vi "Continuous Serial Write and Read_ET_Edited.vi"() -> ()   [LabVIEW 2024]
doc: "This example performs writes and reads on a serial port, as directed by the user. You can press the Write and Read buttons, and change the Read Count, while the example is running.\n\nThe parameters set for the serial port must match the parameters of the connected instrument or device. In this example, the Read Count parameter specifies the number of bytes that the serial port reads. If there were more bytes at the port than the specified number, those bytes would not be read. If there were less bytes at the port than the specified number, you would receive a timeout error.\n\nThis example expands upon the flow control options for XON and XOFF, allowing the user to choose those control characters. Also, the user can enable or disable a termination character. Some devices require a termination character in order to identify the end of command strings. Some devices send a termination character to signify the end of data to be read. This example shows how you can end the Read operation once a termination character is detected in the buffer and/or append a termination character at the end of the Write data."
uses:
  support/Serial - Settings.ctl
  support/Serial - XON-XOFF Characters.ctl
  support/Serial - ASCII Characters.ctl
  <vilib>/Instr/_visa.llb/VISA Configure Serial Port (Instr).vi
panel:
  out "return count":u32
  in  "Stop":bool
  in  "Commands":string[](array[string])=["*RST", "SYST:ZCH ON", "FUNC \"CURR\"", "SYST:ZCOR ON", "CURR:RANG:AUTO ON", "SYST:ZCH OFF", "READ?", ""]
  in  "Termination Character":u8=10 format="%.0x"
  in  "End Write on Termination Character?":bool=TRUE
  in  "Read Count":u32=1000
  out "Response":string
  in  "Write":bool
  in  "Read":bool
  in  "XON/XOFF Characters":T1={"XON"=enum."DC1", "XOFF"=enum."DC3"}
  in  "Serial Settings":T3={"baud rate"=9600, "data bits"=8, "parity"=enum."None", "stop bits"=10, "flow control"=0} {"flow control" items=["None"=0, "XON/XOFF"=1, "RTS/CTS"=2, "DTR/DSR"=4]; "stop bits" items=["1.0"=10, "1.5"=15, "2.0"=20]; "data bits" min=5 max=8 step=1; "baud rate" items=["75"=75, "110"=110, "134"=134, "150"=150, "300"=300, "600"=600, "1200"=1200, "1800"=1800, "2400"=2400, "4800"=4800, "7200"=7200, "9600"=9600, "14400"=14400, "19200"=19200, "28800"=28800, "38400"=38400, "56000"=56000, "57600"=57600, "115200"=115200, "128000"=128000, "230400"=230400]}
  in  "End Read on Termination Character?":bool=TRUE
  in  "VISA resource name":refnum<visa-resource-name>="COM1"
  # "Overview: Demonstrates the use of the VISA functions to write commands to and read responses from a serial instrument continuously in a loop.\nRequirements: NI-VISA Driver\nInstructions:\n1. Run the VI.\n2. Specify a Command and click the Write button.\n3. Read a Response by clicking the Read button.\n4. Click Stop to stop the VI."
  # "0xA is equivalent to a '\\n' character, which is a line feed."
  # "Multi-Commands can be given in one command if seperated by semicolons"
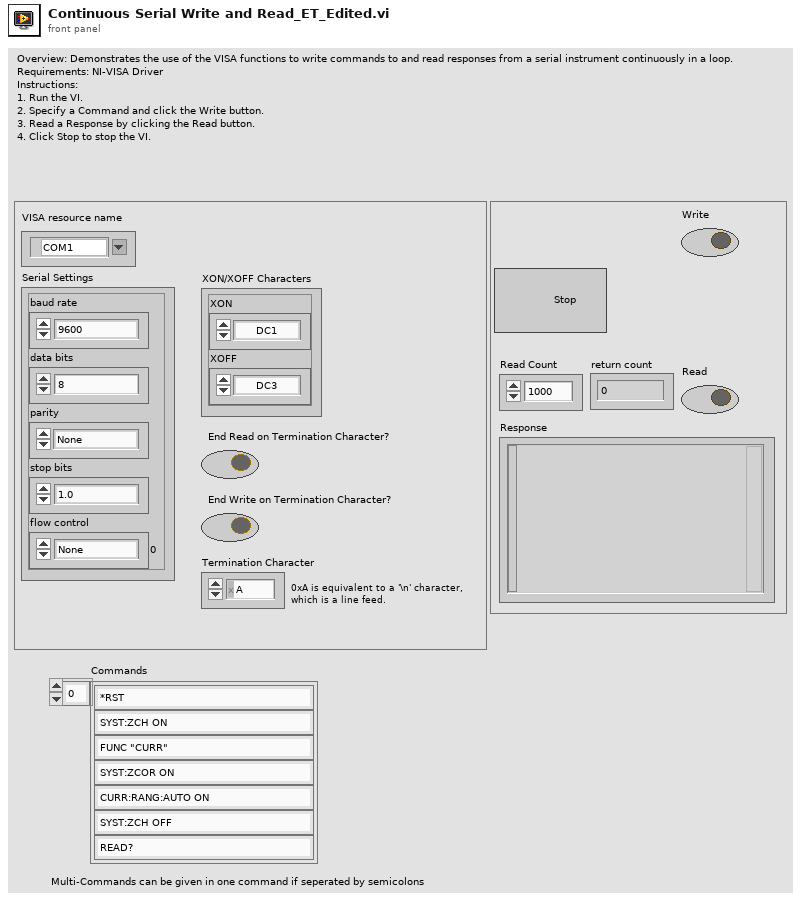
[diagram p1: front panel]
types:
  T1 = typedef "Serial - XON-XOFF Characters.ctl" = cluster{"XON":T2, "XOFF":T2}
  T2 = typedef "Serial - ASCII Characters.ctl" = enum16{"NUL", "SOH", "STX", "ETX", "EOT", "ENQ", "ACK", "BEL", "BS", "HT", "LF", "VT", "FF", "CR", "SO", "SI", "DLE", "DC1", "DC2", "DC3", "DC4", "NAK", "SYN", "ETB", "CAN", "EM", "SUB", "ESC", "FS", "GS", "RS", "US", "SP", "!", "\"", "#", "$", "%", "&", "'", "(", ")", "*", "+", ",", "- (-)", ".", "/", "0", "1", "2", "3", "4", "5", "6", "7", "8", "9", ":", ";", "<", "=", ">", "?", "@", "A", "B", "C", "D", "E", "F", "G", "H", "I", "J", "K", "L", "M", "N", "O", "P", "Q", "R", "S", "T", "U", "V", "W", "X", "Y", "Z", "[", "\\", "]", "^", "_", "`", "a", "b", "c", "d", "e", "f", "g", "h", "i", "j", "k", "l", "m", "n", "o", "p", "q", "r", "s", "t", "u", "v", "w", "x", "y", "z", "{", "|", "}", "~"}
  T3 = typedef "Serial - Settings.ctl" = cluster{"baud rate":u32, "data bits":u16, "parity":enum16{"None", "Odd", "Even", "Mark", "Space"}, "stop bits":u16, "flow control":u16}
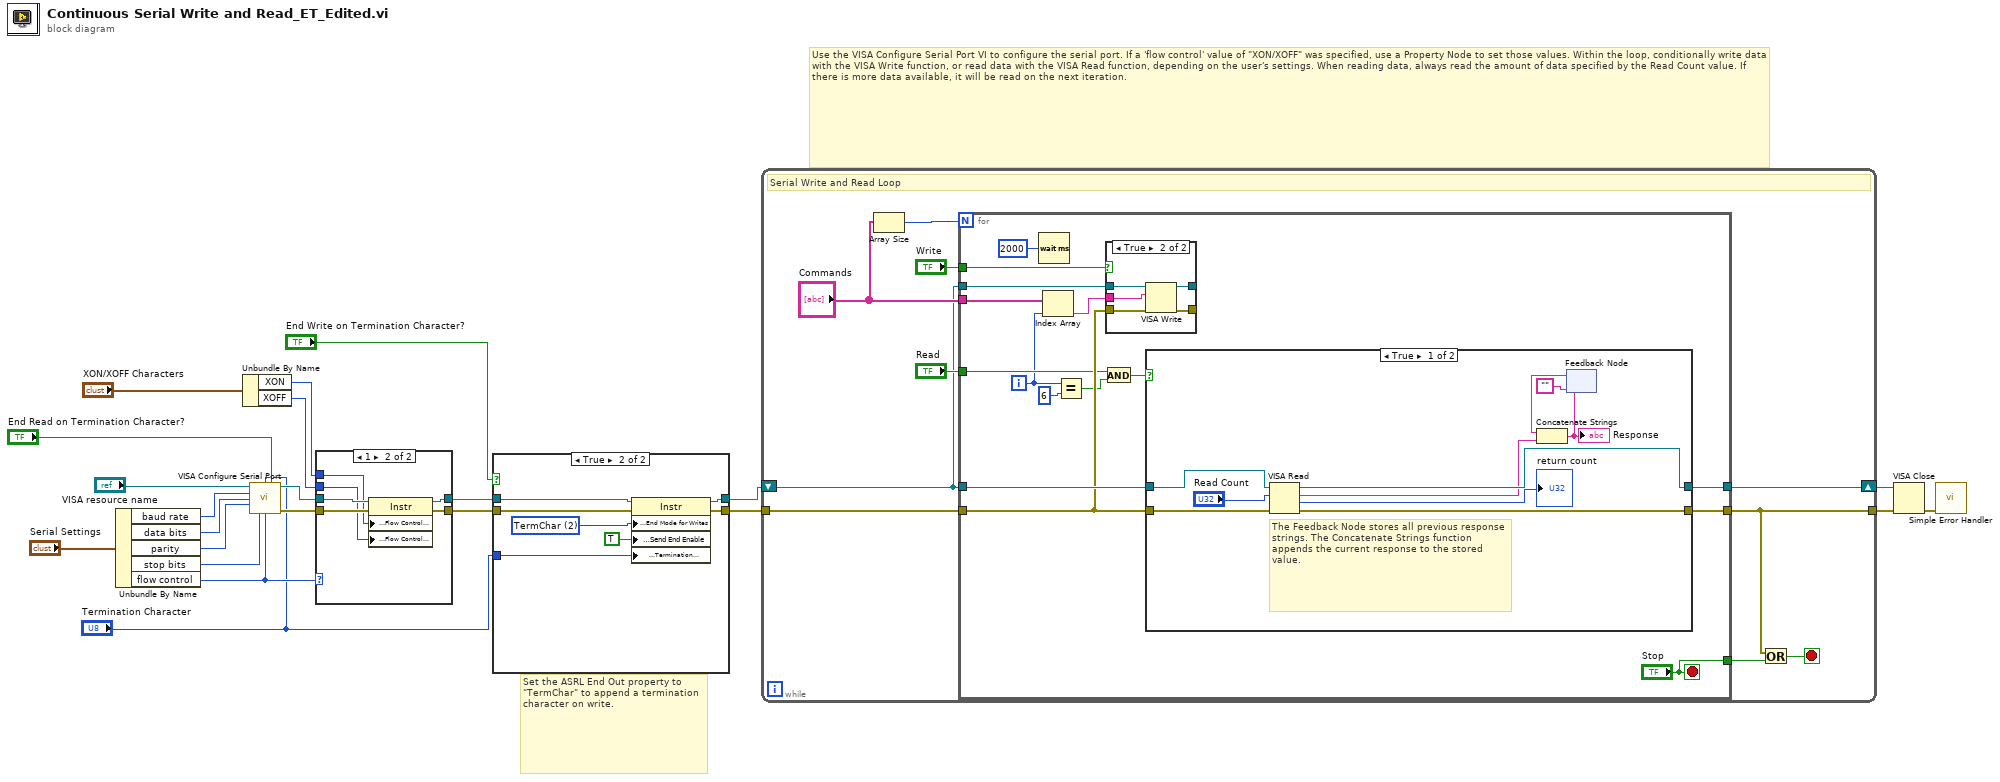
[diagram p0: block diagram]
diagram:
  # "Set the ASRL End Out property to \"TermChar\" to append a termination character on write."
  # "Use the VISA Configure Serial Port VI to configure the serial port. If a 'flow control' value of \"XON/XOFF\" was specified, use a Property Node to set those values. Within the loop, conditionally write data with the VISA Write function, or read data with the VISA Read function, depending on the user's settings. When reading data, always read the amount of data specified by the Read Count value. If there is more data available, it will be read on the next iteration."
  n1 = Unbundle By Name("Serial Settings") -> ("baud rate"=w15:u32, "data bits"=w16:u16, "parity"=w17:enum16{"None", "Odd", "Even", "Mark", "Space"}, "stop bits"=w18:u16, "flow control"=w9:u16)
  n2 = Unbundle By Name("XON/XOFF Characters") -> ("XON"=w8:T2, "XOFF"=w7:T2)
  n3 = call-poly "VISA Configure Serial Port"("VISA resource name"="VISA resource name", "termination char\n(0xA = '\\n' = LF)"="Termination Character", "Enable Termination\nChar (T)"="End Read on Termination Character?", "baud rate (9600)"=w15, "data bits (8)"=w16, "parity (0:none)"=w17, "stop bits (10: 1 bit)"=w18, "flow control (0:none)"=w9) -> ("VISA resource name out"=w19:refnum<visa-resource-name>, "error out"=w20:errorcluster)  [unwired: 2 in, 4 out]
  n4 = case shown="1" w9 {
    tunnel: [w23 w30] -> w6
    tunnel: [w24 w29] -> w4
    tunnel: w20 -> [w23 w28]
    tunnel: w19 -> [w24 w27]
    tunnel: w8 -> [_ w26]
    tunnel: w7 -> [_ w25]
    frame Default {
    }
    frame 1 {
      n5 = property class="Instr"(reference=w27, error in=w28, "Serial Settings:Flow Control XON Character"=w26, "Serial Settings:Flow Control XOFF Character"=w25) -> (reference out=w29:refnum<visa-resource-name>, error out=w30:errorcluster)
    }
  }
  n6 = case shown="True" "End Write on Termination Character?" {
    tunnel: w4 -> [w31 w39]
    tunnel: w6 -> [w32 w38]
    tunnel: [w31 w37] -> w3
    tunnel: [w32 w36] -> w5
    tunnel: "Termination Character" -> [_ w34]
    frame False {
    }
    frame True {
      w35 = u16 2 items=["None", "LastBit", "TermChar", "Break"] ("Serial Settings:Serial End Mode for Writes")
      n7 = property class="Instr"(reference=w39, error in=w38, "Serial Settings:End Mode for Writes"=w35, "Message Based Settings:Send End Enable"=TRUE, "Message Based Settings:Termination Character"=w34) -> (reference out=w37:refnum<visa-resource-name>, error out=w36:errorcluster)
    }
  }
  n8 = while {
    shift-right: [w43] -> w10
    shift-left: w3 -> [w41]
    tunnel: w5 -> [w45]
    tunnel: [w42] -> w11
    stop <- w49 stop-if-true
    # "Serial Write and Read Loop"
    n9 = Array Size(array="Commands") -> (size(s)=w47:i32)
    n10 = for {
      N: w47 -> [_]
      tunnel: "Commands" -> [w64]
      tunnel: "Write" -> [w63]
      tunnel: w41 -> [w62]
      tunnel: w45 -> [w56]
      tunnel: "Read" -> [w55]
      tunnel: [w61] -> w43
      tunnel: [w60] -> w42
      tunnel: w41 -> [w58]
      tunnel: ["Stop"] -> w40
      i -> [w53]
      stop <- "Stop" stop-if-true
      n11 = Wait (ms)(milliseconds to wait=u32 2000) -> ()  [unwired: 1 out]
      n12 = Index Array(array=w64, index=w53) -> (element=w57:string)
      n13 = Equal?(x=w53, y=6) -> (x = y?=w51:bool)
      n14 = And(x=w55, y=w51) -> (x .and. y?=w54:bool)
      n15 = case shown="True" w63 {
        tunnel: w62 -> [w66 w71]
        tunnel: w56 -> [w65 w70]
        tunnel: [w66 w69] -> _
        tunnel: [w65 w68] -> _
        tunnel: w57 -> [_ w67]
        frame False {
        }
        frame True {
          n16 = VISA Write(VISA resource name=w71, write buffer=w67, error in (no error)=w70) -> (VISA resource name out=w69:refnum<visa-resource-name>, error out=w68:errorcluster)  [unwired: 1 out]
        }
      }
      n17 = case shown="True" w54 {
        tunnel: [w79 w83] -> w61
        tunnel: w58 -> [w81 w83]
        tunnel: [w77 w82] -> w60
        tunnel: w56 -> [w80 w82]
        frame True {
          # "The Feedback Node stores all previous response strings. The Concatenate Strings function appends the current response to the stored value."
          n18 = VISA Read(VISA resource name=w81, byte count="Read Count", error in (no error)=w80) -> (VISA resource name out=w79:refnum<visa-resource-name>, read buffer=w76:string, return count=→"return count":u32, error out=w77:errorcluster)
          n19 = feedback #1("") -> (w75:string)
          n20 = Concatenate Strings(w75, w76) -> (w74:string)
          "Response" <- w74
          n21 = feedback-in #1(w74) -> ()
        }
        frame False {
        }
      }
    }
    n22 = Or(x=w42, y=w40) -> (x .or. y?=w49:bool)
  }
  n23 = VISA Close(VISA resource name=w10, error in (no error)=w11) -> (error out=w12:errorcluster)
  n24 = call <vilib>:"Simple Error Handler.vi"("error in (no error)"=w12) -> ()  [unwired: 1 in, 8 out]
